vi "Interpolate power.vi"(9 "Point below":cluster{"Frequency":dbl, "Power":dbl}, 10 "Frequency (GHz)":dbl, 11 "Point above":cluster{"Frequency":dbl, "Power":dbl}) -> (3 "Power (mW)":dbl)   [LabVIEW 2015, in "Power control.lvclass"]
uses:
  Power control.lvclass
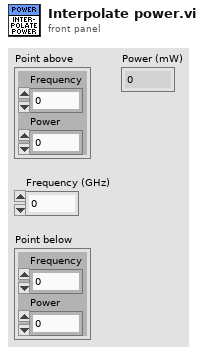
[diagram p1: front panel]
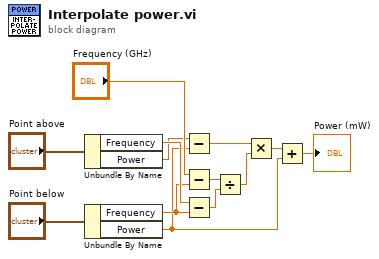
[diagram p0: block diagram]
diagram:
  n1 = Unbundle By Name("Point above") -> ("Frequency"=w10:dbl, "Power"=w5:dbl)
  n2 = Unbundle By Name("Point below") -> ("Frequency"=w9:dbl, "Power"=w2:dbl)
  n3 = Subtract(x=w5, y=w2) -> (x-y=w4:dbl)
  n4 = Subtract(x="Frequency (GHz)", y=w9) -> (x-y=w7:dbl)
  n5 = Subtract(x=w10, y=w9) -> (x-y=w8:dbl)
  n6 = Divide(x=w7, y=w8) -> (x/y=w6:dbl)
  n7 = Multiply(x=w4, y=w6) -> (x*y=w3:dbl)
  n8 = Add(x=w3, y=w2) -> (x+y=→"Power (mW)":dbl)
